vi "New.vi"(8 "error in (no error)":errorcluster, 11 "icon path":path) -> (0 "error out":errorcluster, 3 "icon out":refnum<class "icon.lvclass">)   [LabVIEW 2009, in "icon.lvclass"]
uses:
  icon.lvclass
  icon.lvclass/icon.ctl
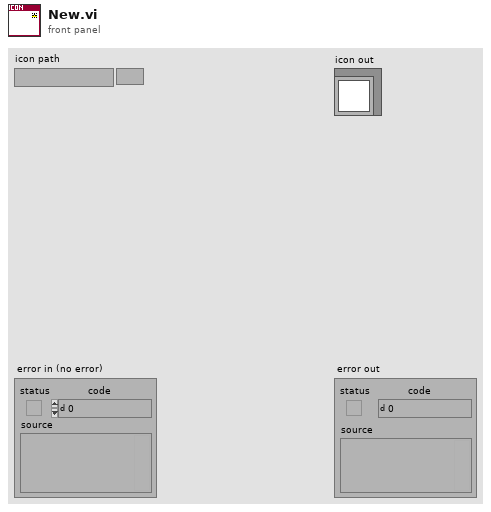
[diagram p1: front panel]
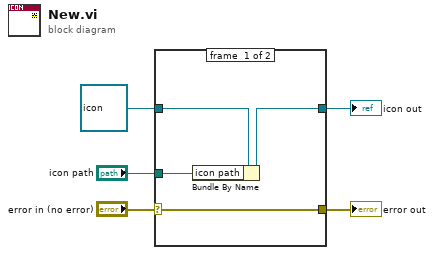
[diagram p0: block diagram]
diagram:
  n1 = case shown="No Error" "error in (no error)" {
    selector: "error in (no error)" -> [w8 w11]
    tunnel: [w8 w11] -> w2
    tunnel: [w7 w10] -> w4
    tunnel: refnum<class "icon.lvclass"> refnum ("icon in") -> [w9 w10]
    tunnel: "icon path" -> [w6 _]
    frame #0 {
      n2 = Bundle By Name(cluster=w9, "icon path"=w6) -> (w7:refnum<class "icon.lvclass">)
    }
    frame #1 {
    }
  }
  "icon out" <- w4
  "error out" <- w2
